vi "Main_Manual_Control.vi"() -> ()   [LabVIEW 2020]
uses:
  States.ctl
  <vilib>/Utility/file.llb/Read Delimited Spreadsheet (I64).vi
  <vilib>/Instr/_visa.llb/VISA Configure Serial Port (Serial Instr).vi
panel:
  in  "Manual Mode":bool
  in  "Tab Control":enum32{"Control", "Debug"}(tab)
  out "Power":dynamicdata(graph)
  in  "Power DAQ":bool
  in  "Log DAQ":bool
  out "Target INC":u16 max=12 step=1
  out "STEP":i32
  out "Target MPH":u16 max=12 step=1
  out "stopping":bool
  in  "Serial Port":refnum<visa-resource-name>="COM8"
  in  "Manual Stop":bool
  in  "TestScript":path=path "C:/LabView Computer Backup SEAL2788/DonP_TRM500/FootTimeInc.txt"
  out "MPH READ":u8
  out "INC READ":u8
  out "PD READ":u8
  out "Speed Changed":bool
  out "Inc Changed":bool
  in  "MPH UP":bool
  in  "MPH DOWN":bool
  in  "INC UP":bool
  in  "INC DOWN":bool
  out "Com Error":errorcluster
  out "Control Error":errorcluster
  out "speed":u16[](array[numeric])
  out "time":u16[](array[numeric])
  out "incline":u16[](array[numeric])
  out "dwell":u16[](array[numeric])
  out "FootPath":path
  out "read buffer":string
  out "Send Buffer":string
  out "Last Speed Sent":string
  out "Last Inc Sent":string
  out "FootPathRef":refnum<file>
  out "input lines":i32
  out "Next Inc":u16
  out "Next Duration":u16
  out "Next MPH":u16
  out "Time Left":u32
  out "Missed Msg":u16
  out "Next Cmd":enum16{"getParm", "inc", "mph", "err"}(ring)
  out "Next Com State":enum16{"Initialize", "Send", "Receive", "Error"}(ring)=enum."Receive"
  out "Next Control State":T1
  # "Control Panel"
  # "Debug Panel"
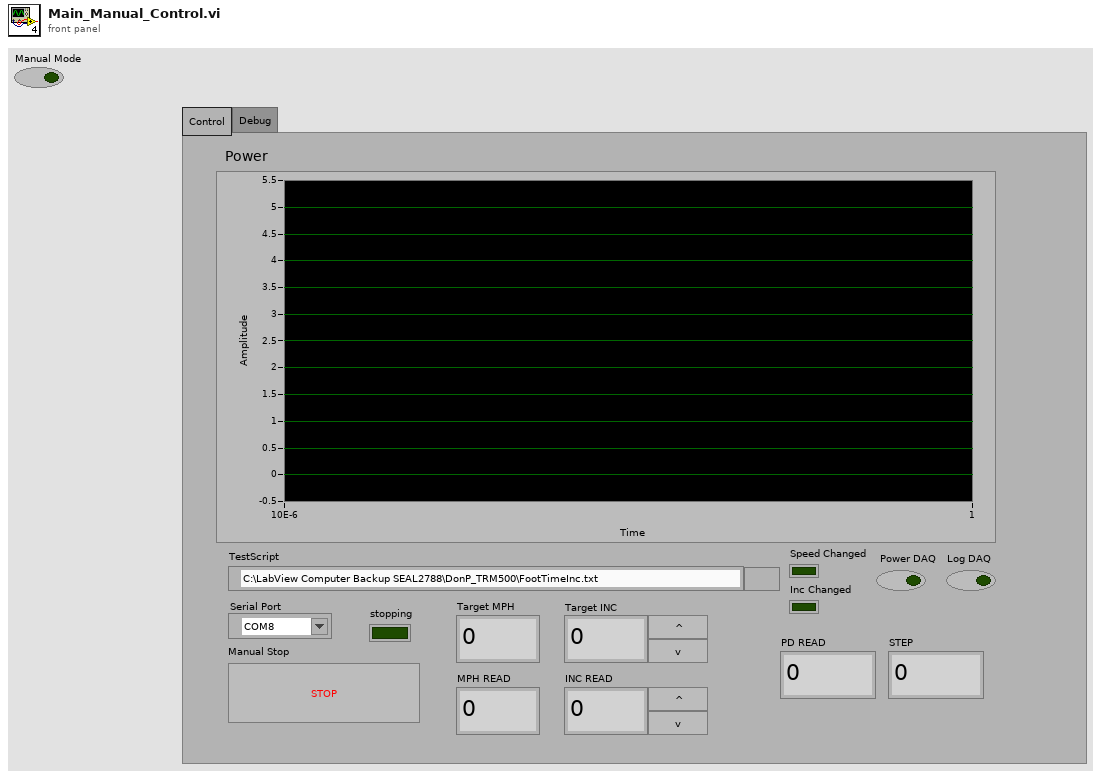
[diagram p1: front panel]
types:
  T1 = typedef "States.ctl" = enum16{"Initialize", "SetTargets", "WaitforMPH", "Dwell", "CheckTiming"}
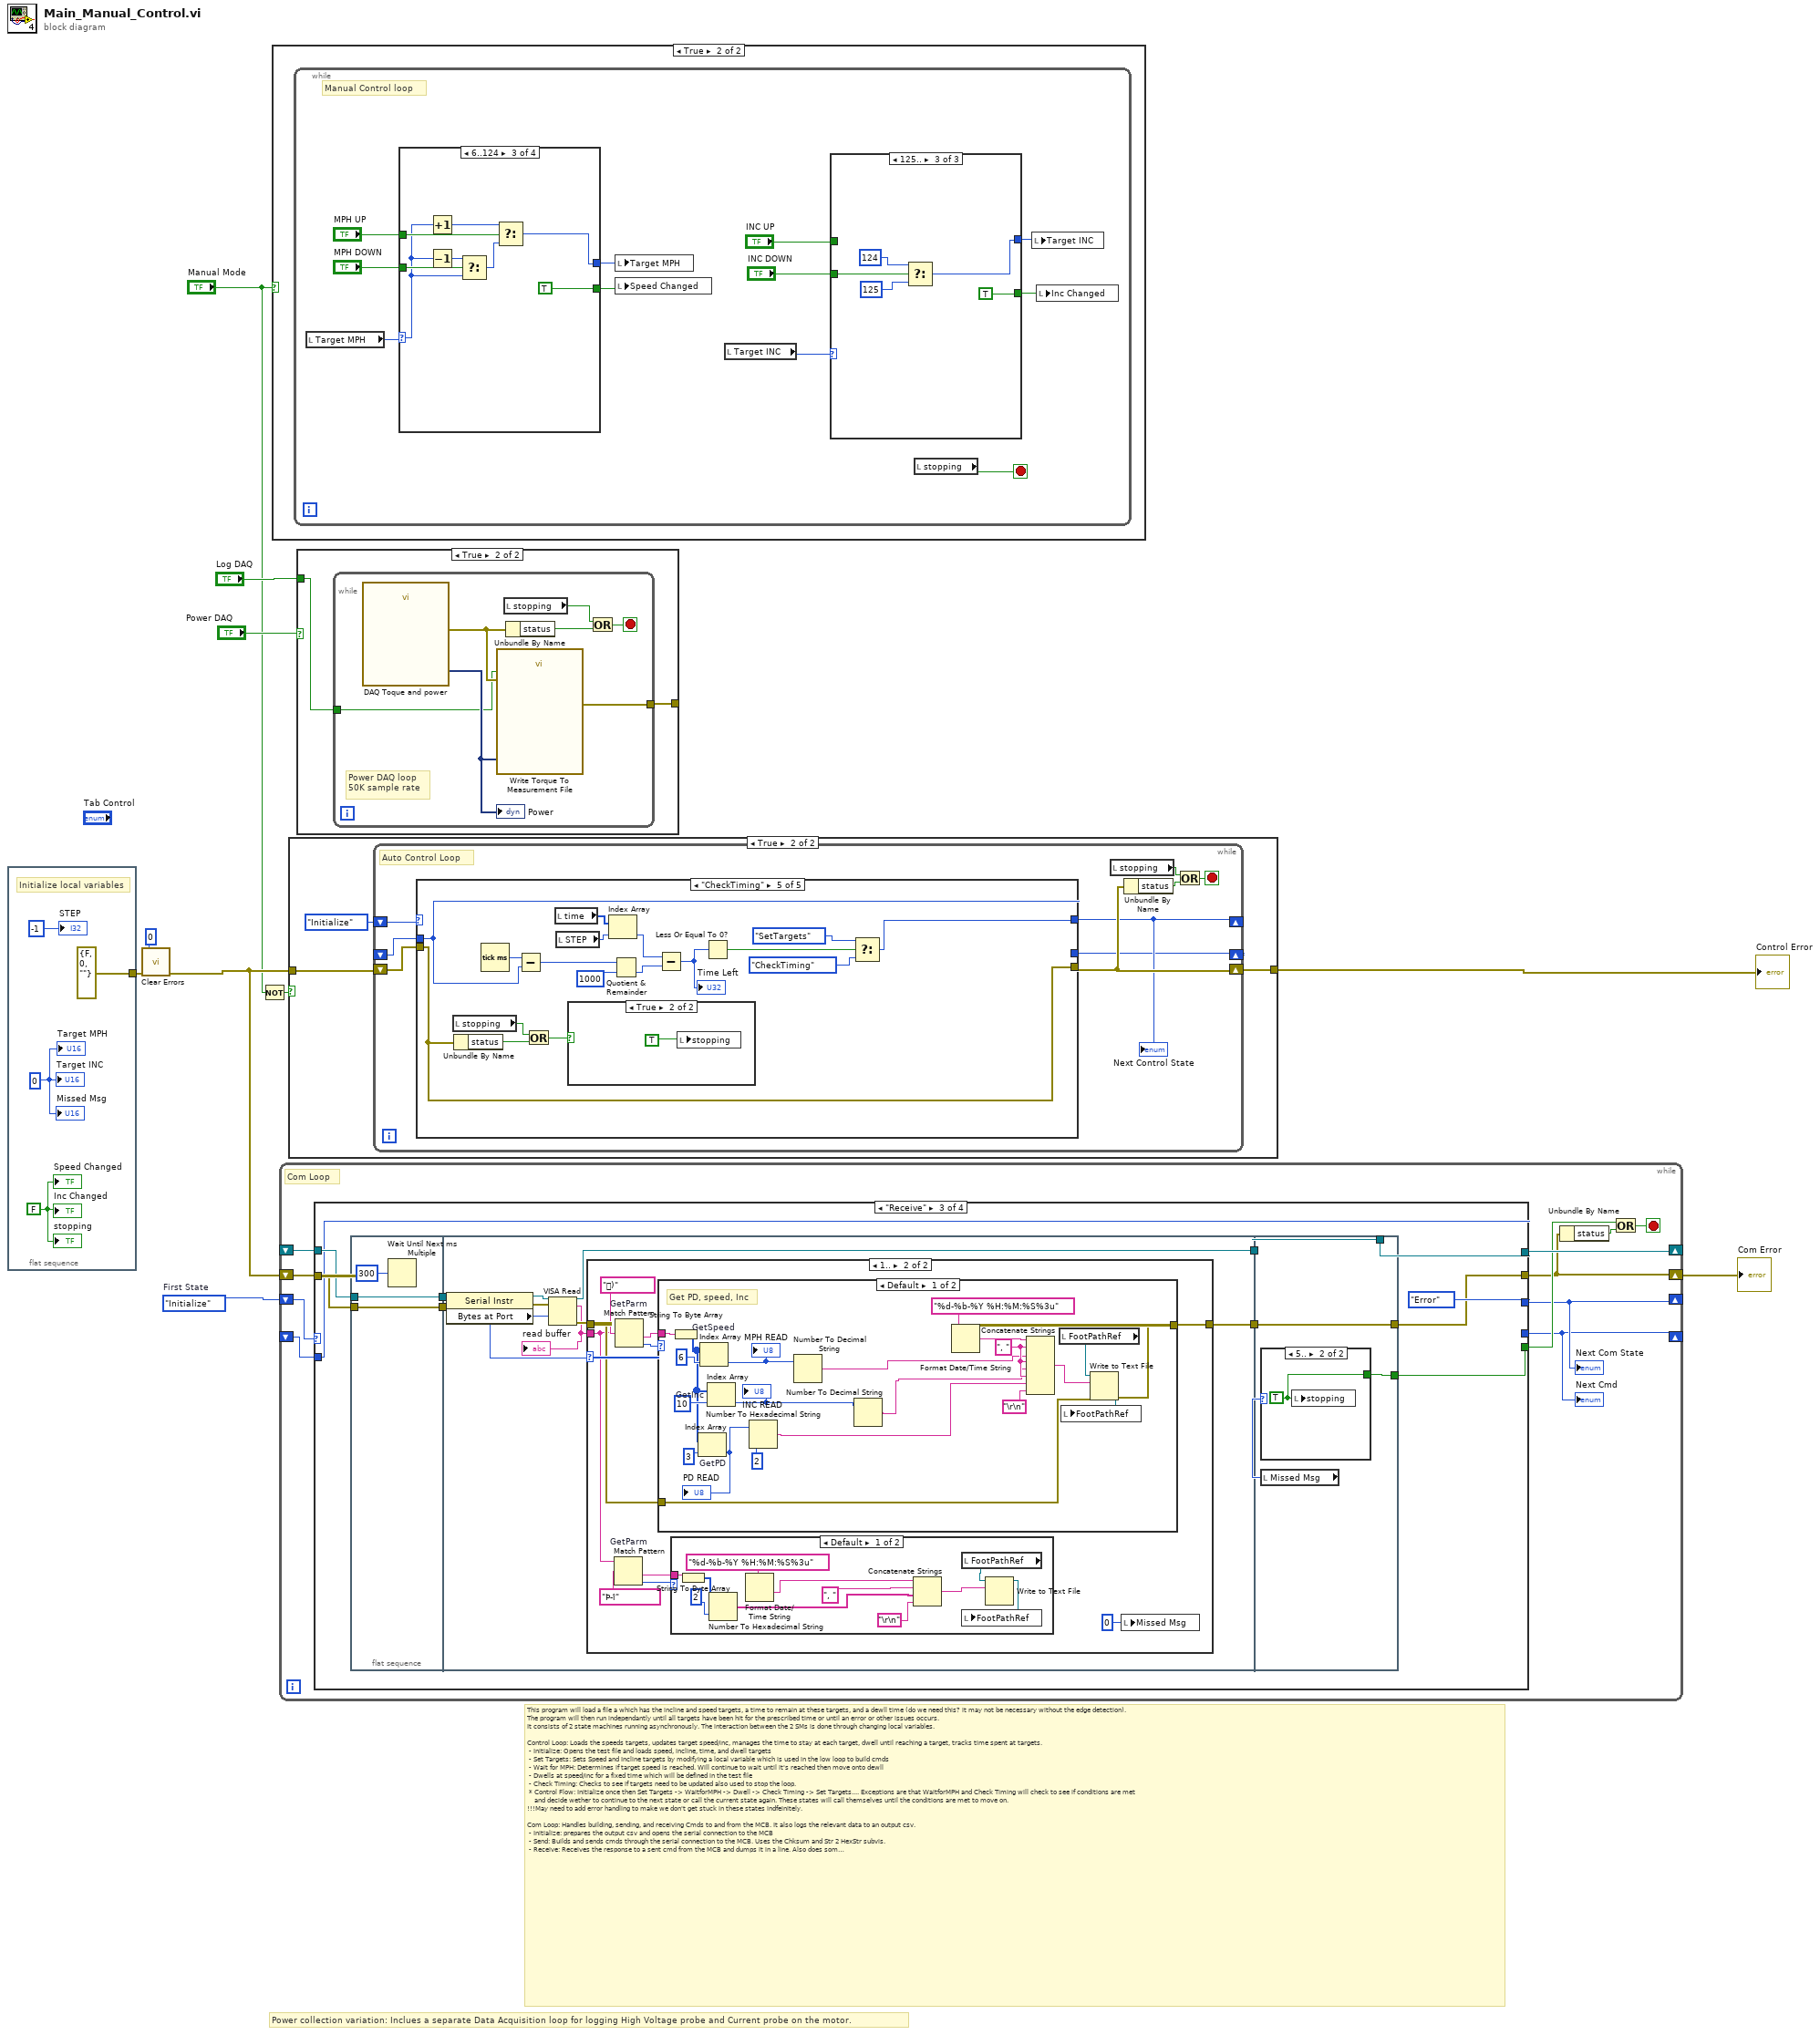
[diagram p0: block diagram]
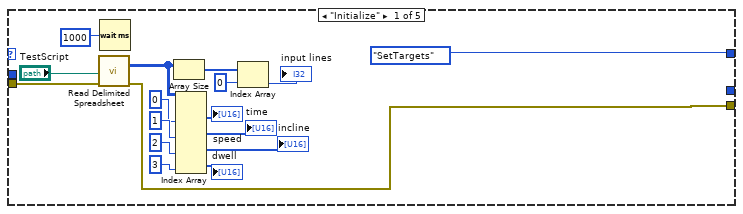
[diagram p3: hidden frame]
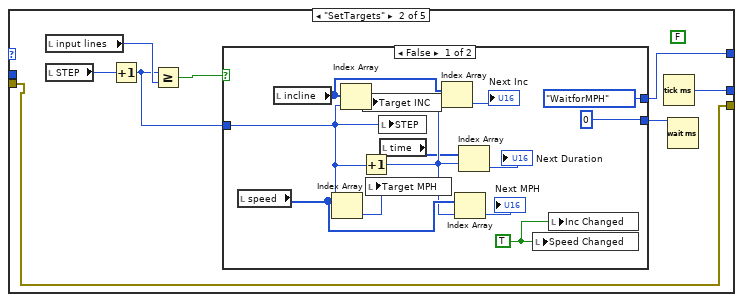
[diagram p4: hidden frame]
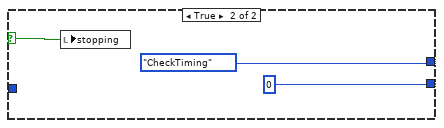
[diagram p5: hidden frame]
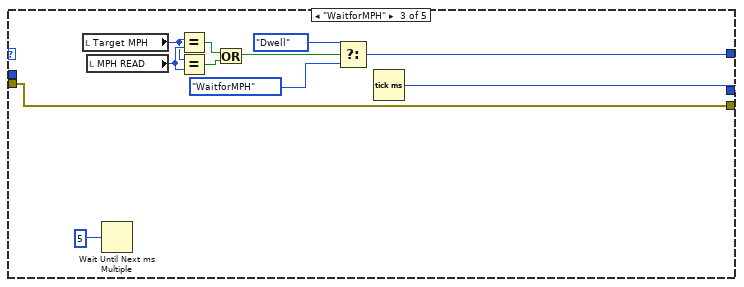
[diagram p6: hidden frame]
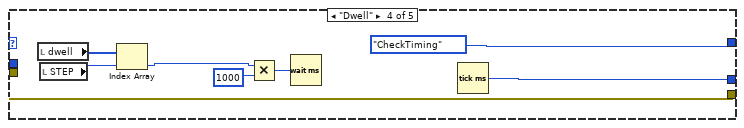
[diagram p7: hidden frame]
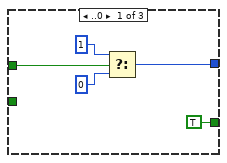
[diagram p10: hidden frame]
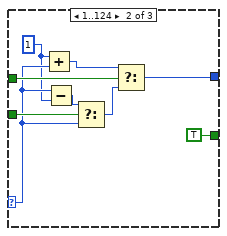
[diagram p11: hidden frame]
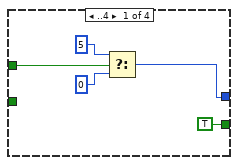
[diagram p12: hidden frame]
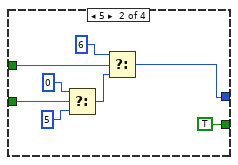
[diagram p13: hidden frame]
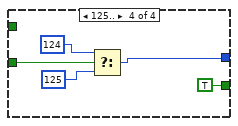
[diagram p14: hidden frame]
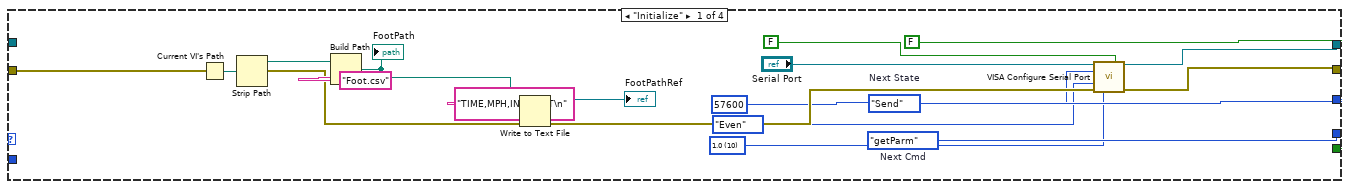
[diagram p16: hidden frame]
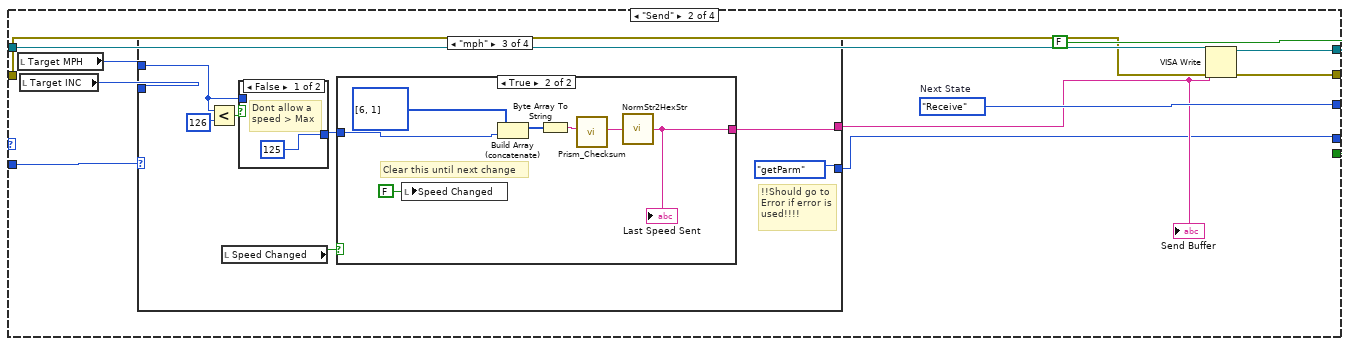
[diagram p17: hidden frame]
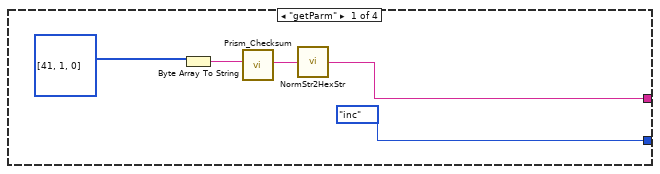
[diagram p18: hidden frame]
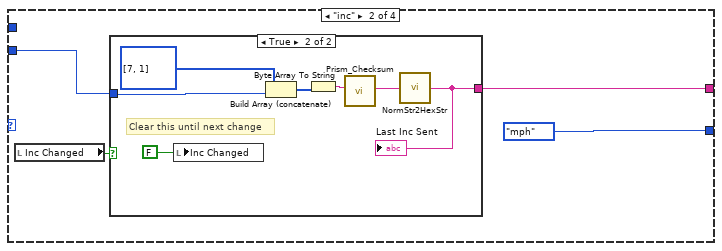
[diagram p19: hidden frame]
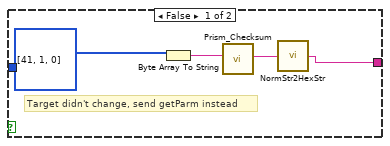
[diagram p20: hidden frame]
diagram:
  w10 = enum16{"Initialize", "Send", "Receive", "Error"}."Initialize"  # First State
  # "Power collection variation: Inclues a separate Data Acquisition loop for logging High Voltage probe and Current probe on the motor."
  # "This program will load a file a which has the incline and speed targets, a time to remain at these targets, and a dewll time (do we need this? it may not be necessary without the edge detection).\nThe program will then run independantly until all targets have been hit for the prescribed time or until an error or other issues occurs.\nIt consists of 2 state machines running asynchronously. The interaction between the 2 SMs is done through changing local variables.\n\nControl Loop: Loads the speeds targets, updates target speed/inc, manages the time to stay at each target, dwell until reaching a target, tracks time spent at targets. \n - Initialize: Opens the test file and loads speed, incline, time, and dwell targets \n - Set Targets: Sets Speed and Incline targets by modifying a local variable which is used in the low loop to build cmds \n - Wait for MPH: Determines if target speed is reached. Will continue to wait until it's reached then move onto dewll\n - Dwells at speed/inc for a fixed time which will be defined in the test file\n - Check Timing: Checks to see if targets need to be updated also used to stop the loop.\n * Control Flow: Initialize once then Set Targets -> WaitforMPH -> Dwell -> Check Timing -> Set Targets.... Exceptions are that WaitforMPH and Check Timing will check to see if conditions are met\n    and decide wether to continue to the next state or call the current state again. These states will call themselves until the conditions are met to move on. \n!!!May need to add error handling to make we don't get stuck in these states indfeinitely.\n\nCom Loop: Handles building, sending, and receiving Cmds to and from the MCB. It also logs the relevant data to an output csv.\n - Initialize: prepares the output csv and opens the serial connection to the MCB\n - Send: Builds and sends cmds through the serial connection to the MCB. Uses the Chksum and Str 2 HexStr subvis. \n - Receive: Receives the response to a sent cmd from the MCB and dumps it in a line. Also does some analysis of the response to determine current  Speed/inc/person detect\n - Error:  Stops the program. This handles labview errors and will stop the program when one is encounted. It also handles stopping when reaching the end of a test \n * Com Flow: nitialize once then Send -> Receive -> Error -> Send...\n * Send flow: GetParm -> Inc -> MPH -> GetParm etc. Exception is that it will check first to see if the target changed and if it hasn't will send getParm Instead\n!!!May need to add error handling in which case the flow should be GetParm -> MPH -> Inc -> Err -> GetParm....\n\nFiles:\n1 input file which contains the test script to run. Format: Speed, Time, Inc, Dwell. Time = time to stay at target speed/inc. Dwell = a fixed time to wait after reaching targets and before starting the Time counter. This is used to make sure the speed stablizes before starting the Time counter.\n1 output file which contains Timestamp, Speed, Incline, and a flag for if person is detected (0 = No, 1 = Yes). Format: TIME,MPH,INC,FOOT"
  n1 = flat-sequence {
    tunnel: [errorcluster {"status"=FALSE, "code"=0, "source"=""} ("error constant")] -> w7
    frame #0 {
      w12 = FALSE ("Inc Changed")
      w11 = u16 0 ("MPH")
      # "Initialize local variables"
      "stopping" <- w12
      "Target MPH" <- w11
      "STEP" <- -1 ("step")
      "Target INC" <- w11
      "Speed Changed" <- w12
      "Inc Changed" <- w12
      "Missed Msg" <- w11
    }
  }
  n2 = call <vilib>:"Clear Errors.vi"("error in (no error)"=w7, "specific error code to clear (0: all)"=0) -> ("error out"=w6:errorcluster)  [unwired: 4 in, 1 out]
  n3 = Not(x="Manual Mode") -> (.not. x?=w1:bool)
  n4 = case shown="True" "Manual Mode" {
    frame False {
    }
    frame True {
      n5 = while {
        stop <- w25 stop-if-true
        # "Manual Control loop"
        n6 = local read "Target MPH"() -> (w20:u16)
        n7 = case shown="6..124" w20 {
          selector: w20 -> [_ _ w61 _]
          tunnel: "MPH UP" -> [w49 w57 w65 _]
          tunnel: "MPH DOWN" -> [_ w54 w63 w70]
          tunnel: [w46 w51 w59 w67] -> w18
          tunnel: [TRUE TRUE TRUE TRUE] -> w16
          frame ..4 {
            n8 = Select(t=5 ("MPH"), s=w49, f=0 ("MPH")) -> (s? t:f=w46:i32)
          }
          frame 5 {
            n9 = Select(t=0 ("MPH"), s=w54, f=5 ("MPH")) -> (s? t:f=w55:i32)
            n10 = Select(t=6 ("MPH"), s=w57, f=w55) -> (s? t:f=w51:i32)
          }
          frame 6..124 {
            n11 = Increment(x=w61) -> (x+1=w60:u16)
            n12 = Decrement(x=w61) -> (x-1=w62:u16)
            n13 = Select(t=w62, s=w63, f=w61) -> (s? t:f=w64:u16)
            n14 = Select(t=w60, s=w65, f=w64) -> (s? t:f=w59:u16)
          }
          frame 125.. {
            n15 = Select(t=124 ("MPH"), s=w70, f=125) -> (s? t:f=w67:i32)
          }
        }
        n16 = local write "Target MPH"(w18) -> ()
        n17 = local write "Speed Changed"(w16) -> ()
        n18 = local read "Target INC"() -> (w19:u16)
        n19 = case shown="125.." w19 {
          selector: w19 -> [_ w35 _]
          tunnel: "INC UP" -> [w30 w39 _]
          tunnel: "INC DOWN" -> [_ w37 w44]
          tunnel: [w27 w32 w41] -> w17
          tunnel: [TRUE TRUE TRUE] -> w15
          frame ..0 {
            n20 = Select(t=1 ("MPH"), s=w30, f=0 ("MPH")) -> (s? t:f=w27:i32)
          }
          frame 1..124 {
            w34 = 1
            n21 = Add(x=w34, y=w35) -> (x+y=w36:i32)
            n22 = Subtract(x=w35, y=w34) -> (x-y=w33:i32)
            n23 = Select(t=w33, s=w37, f=w35) -> (s? t:f=w38:i32)
            n24 = Select(t=w36, s=w39, f=w38) -> (s? t:f=w32:i32)
          }
          frame 125.. {
            n25 = Select(t=124 ("MPH"), s=w44, f=125) -> (s? t:f=w41:i32)
          }
        }
        n26 = local read "stopping"() -> (w25:bool)
        n27 = local write "Target INC"(w17) -> ()
        n28 = local write "Inc Changed"(w15) -> ()
      }
    }
  }
  n29 = while {
    shift-right: [w75] -> w9
    shift-left: w6 -> [w81]
    shift-right: [w78] -> _
    shift-left: _ -> [w80]
    shift-right: [w72] -> _
    shift-left: w10 -> [w79]
    shift-right: [w71] -> _
    shift-left: _ -> [w77]
    stop <- w74 stop-if-true
    # "Com Loop"
    n30 = case shown="\"Receive\"" w79 {
      tunnel: w81 -> [w87 w101 w164 w234]
      tunnel: w80 -> [_ w108 w166 w232]
      tunnel: [w97 w110 w160 w231] -> w78
      tunnel: [w96 w109 w159 w233] -> w75
      tunnel: [w93 w104 enum16{"Initialize", "Send", "Receive", "Error"}."Error" enum16{"Initialize", "Send", "Receive", "Error"}."Send"] -> w72
      tunnel: [w95 w102 w163 w239] -> w71
      tunnel: w77 -> [_ w100 w163 w239]
      tunnel: [FALSE FALSE w156 w235] -> w76
      frame "Initialize" {
        w82 = u16 10 items=["1.0"=10, "1.5"=15, "2.0"=20] ("stop bits (10: 1 bit)")
        w93 = enum16{"Initialize", "Send", "Receive", "Error"}."Send"  # Next State
        w95 = enum16{"getParm", "inc", "mph", "err"}."getParm"  # Next Cmd
        n31 = Current VI's Path() -> (path=w92:path)
        n32 = Strip Path(path=w92) -> (stripped path=w91:path)  [unwired: 1 out]
        n33 = Build Path(base path=w91, name or relative path="Foot.csv") -> (appended path=w88:path)
        "FootPath" <- w88
        n34 = Write to Text File(file (use dialog)=w88, text="TIME,MPH,INC,FOOT\n", error in=w87) -> (refnum out=→"FootPathRef":refnum<file>, error out=w86:errorcluster)  [unwired: 1 in, 1 out]
        n35 = call-poly "VISA Configure Serial Port"("VISA resource name"="Serial Port", "Enable Termination\nChar (T)"=FALSE ("Enable Termination\nChar (T)"), "baud rate (9600)"=u32 57600, "parity (0:none)"=enum16{"None", "Odd", "Even", "Mark", "Space"}."Even", "error in (no error)"=w86, "stop bits (10: 1 bit)"=w82) -> ("VISA resource name out"=w97:refnum<visa-resource-name>, "error out"=w96:errorcluster)  [unwired: 8 in]
      }
      frame "Send" {
        w104 = enum16{"Initialize", "Send", "Receive", "Error"}."Receive"  # Next State
        n36 = local read "Target MPH"() -> (w106:u16)
        n37 = local read "Target INC"() -> (w105:u16)
        n38 = case shown="\"mph\"" w100 {
          tunnel: w106 -> [_ _ w132 _]
          tunnel: w105 -> [_ w119 _ _]
          tunnel: [w111 w118 w136 w152] -> w103
          tunnel: [enum16{"getParm", "inc", "mph", "err"}."inc" enum16{"getParm", "inc", "mph", "err"}."mph" enum16{"getParm", "inc", "mph", "err"}."getParm" enum16{"getParm", "inc", "mph", "err"}."getParm"] -> w102
          frame "getParm" {
            n39 = Byte Array To String(unsigned byte array=u8[] [41, 1, 0]) -> (string=w113:string)
            n40 = call "Prism_Checksum.vi"("ID +DB+ Data"=w113) -> ("Full Cmd"=w112:string)  [unwired: 10 in]
            n41 = call "NormStr2HexStr.vi"("string"=w112) -> ("hex string"=w111:string)
          }
          frame "inc" {
            n42 = local read "Inc Changed"() -> (w116:bool)
            n43 = case shown="True" w116 {
              tunnel: w119 -> [_ w127]
              tunnel: [w120 w125] -> w118
              frame False {
                # "Target didn't change, send getParm instead"
                n44 = Byte Array To String(unsigned byte array=u8[] [41, 1, 0]) -> (string=w122:string)
                n45 = call "Prism_Checksum.vi"("ID +DB+ Data"=w122) -> ("Full Cmd"=w121:string)  [unwired: 10 in]
                n46 = call "NormStr2HexStr.vi"("string"=w121) -> ("hex string"=w120:string)
              }
              frame True {
                # "Clear this until next change"
                n47 = local write "Inc Changed"(FALSE ("Value Changed")) -> ()
                n48 = Build Array (concatenate)(u8[] [7, 1] ("unsigned byte array"), w127) -> (w126:u16[])
                n49 = Byte Array To String(unsigned byte array=w126) -> (string=w129:string)
                n50 = call "Prism_Checksum.vi"("ID +DB+ Data"=w129) -> ("Full Cmd"=w130:string)  [unwired: 10 in]
                n51 = call "NormStr2HexStr.vi"("string"=w130) -> ("hex string"=w125:string)
                "Last Inc Sent" <- w125
              }
            }
          }
          frame "mph" {
            # "!!Should go to\nError if error is\nused!!!!"
            n52 = Less?(x=w132, y=u16 126) -> (x < y?=w134:bool)
            n53 = local read "Speed Changed"() -> (w135:bool)
            n54 = case shown="False" w134 {
              tunnel: w132 -> [_ w139]
              tunnel: [u16 125 ("Target MPH") w139] -> w131
              frame False {
                # "Dont allow a\nspeed > Max"
              }
              frame True {
              }
            }
            n55 = case shown="True" w135 {
              tunnel: [w140 w147] -> w136
              tunnel: w131 -> [_ w145]
              frame False {
                # "Target didn't change, send getParm instead"
                n56 = Byte Array To String(unsigned byte array=u8[] [41, 1, 0]) -> (string=w142:string)
                n57 = call "Prism_Checksum.vi"("ID +DB+ Data"=w142) -> ("Full Cmd"=w141:string)  [unwired: 10 in]
                n58 = call "NormStr2HexStr.vi"("string"=w141) -> ("hex string"=w140:string)
              }
              frame True {
                # "Clear this until next change"
                n59 = local write "Speed Changed"(FALSE ("Value Changed")) -> ()
                n60 = Build Array (concatenate)(u8[] [6, 1] ("unsigned byte array"), w145) -> (w146:u16[])
                n61 = Byte Array To String(unsigned byte array=w146) -> (string=w149:string)
                n62 = call "Prism_Checksum.vi"("ID +DB+ Data"=w149) -> ("Full Cmd"=w150:string)  [unwired: 10 in]
                n63 = call "NormStr2HexStr.vi"("string"=w150) -> ("hex string"=w147:string)
                "Last Speed Sent" <- w147
              }
            }
          }
          frame "err" {
            # "!!Not in used currently. DELETE this if implemented!!!"
            # "!!!!Add logic to\nhandle/ clear erros!!!!!!"
            n64 = Byte Array To String(unsigned byte array=u8[] [30, 1, 0]) -> (string=w154:string)
            n65 = call "Prism_Checksum.vi"("ID +DB+ Data"=w154) -> ("Full Cmd"=w155:string)  [unwired: 10 in]
            n66 = call "NormStr2HexStr.vi"("string"=w155) -> ("hex string"=w152:string)
          }
        }
        "Send Buffer" <- w103
        n67 = VISA Write(VISA resource name=w108, write buffer=w103, error in (no error)=w101) -> (VISA resource name out=w110:refnum<visa-resource-name>, error out=w109:errorcluster)  [unwired: 1 out]
      }
      frame "Receive" {
        n68 = flat-sequence {
          tunnel: w166 -> [w168]
          tunnel: w164 -> [w167]
          tunnel: [w168] -> w162
          tunnel: [w167] -> w161
          tunnel: w162 -> [w178]
          tunnel: w161 -> [w177]
          tunnel: [w170] -> w158
          tunnel: [w174] -> w157
          tunnel: [w227] -> w159
          tunnel: [w228] -> w160
          tunnel: w158 -> [w228]
          tunnel: w157 -> [w227]
          tunnel: [w225] -> w156
          frame #0 {
            n69 = Wait Until Next ms Multiple(millisecond multiple=u32 300) -> ()  [unwired: 1 out]
          }
          frame #1 {
            n70 = property class="Serial Instr"(reference=w178, error in=w177) -> (reference out=w175:refnum<visa-resource-name>, error out=w176:errorcluster, "Bytes at Port"=w173:u32)
            n71 = VISA Read(VISA resource name=w175, byte count=w173, error in (no error)=w176) -> (VISA resource name out=w170:refnum<visa-resource-name>, read buffer=w171:string, error out=w172:errorcluster)  [unwired: 1 out]
            "read buffer" <- w171
            n72 = case shown="1.." w173 {
              tunnel: [w181 w188] -> w174
              tunnel: w172 -> [w181 w187]
              tunnel: w171 -> [_ w186]
              frame 0 {
                n73 = local read "Missed Msg"() -> (w180:u16)
                n74 = Increment(x=w180) -> (x+1=w179:u16)
                n75 = local write "Missed Msg"(w179) -> ()
              }
              frame 1.. {
                n76 = Match Pattern "GetParm"(string=w186, regular expression="Þ­î") -> (after substring=w183:string, offset past match=w184:i32)  [unwired: 1 in, 2 out]
                n77 = Match Pattern "GetParm"(string=w186, regular expression="ޭ)") -> (after substring=w190:string, offset past match=w189:i32)  [unwired: 1 in, 2 out]
                n78 = case shown="Default" w189 {
                  tunnel: w190 -> [w204 _]
                  tunnel: [w217 w224] -> w188
                  tunnel: w187 -> [w212 w224]
                  frame Default {
                    w211 = ", "
                    # "Get PD, speed, Inc"
                    n79 = String To Byte Array(string=w204) -> (unsigned byte array=w220:u8[])
                    n80 = Index Array "GetPD"(array=w220, index=3) -> (element=w214:u8)
                    "PD READ" <- w214
                    n81 = Index Array "GetSpeed"(array=w220, index=6) -> (element=w206:u8)
                    "MPH READ" <- w206
                    n82 = Index Array "GetInc"(array=w220, index=10) -> (element=w205:u8)
                    "INC READ" <- w205
                    n83 = Number To Hexadecimal String(1:i16 2 ("width (-)"), 2:w214) -> (0:w209:string)
                    n84 = Number To Decimal String(number=w206) -> (decimal integer string=w208:string)  [unwired: 1 in]
                    n85 = Number To Decimal String(number=w205) -> (decimal integer string=w207:string)  [unwired: 1 in]
                    n86 = Format Date/Time String(time format string (%c)="%d-%b-%Y %H:%M:%S%3u") -> (date/time string=w215:string)  [unwired: 2 in]
                    n87 = Concatenate Strings(w215, w211, w208, w211, w207, w211, w209, "\r\n") -> (w218:string)
                    n88 = local read "FootPathRef"() -> (w216:refnum<file>)
                    n89 = Write to Text File(file (use dialog)=w216, text=w218, error in=w212) -> (refnum out=w210:refnum<file>, error out=w217:errorcluster)  [unwired: 1 in, 1 out]
                    n90 = local write "FootPathRef"(w210) -> ()
                  }
                  frame -1 {
                  }
                }
                n91 = case shown="Default" w184 {
                  tunnel: w183 -> [w197 _]
                  frame Default {
                    n92 = String To Byte Array(string=w197) -> (unsigned byte array=w195:u8[])
                    n93 = Number To Hexadecimal String(1:i16 2 ("width (-)"), 2:w195) -> (0:w192:string[])
                    n94 = Format Date/Time String(time format string (%c)="%d-%b-%Y %H:%M:%S%3u") -> (date/time string=w199:string)  [unwired: 2 in]
                    n95 = Concatenate Strings(w199, ", ", w192, "\r\n") -> (w198:string)
                    n96 = local read "FootPathRef"() -> (w202:refnum<file>)
                    n97 = Write to Text File(file (use dialog)=w202, text=w198) -> (refnum out=w201:refnum<file>)  [unwired: 2 in, 2 out]
                    n98 = local write "FootPathRef"(w201) -> ()
                  }
                  frame -1 {
                  }
                }
                n99 = local write "Missed Msg"(u16 0 ("Missed Msg")) -> ()
              }
            }
          }
          frame #2 {
            n100 = local read "Missed Msg"() -> (w226:u16)
            n101 = case shown="5.." w226 {
              tunnel: [FALSE ("stopping") w230] -> w225
              frame ..4 {
              }
              frame 5.. {
                w230 = TRUE ("stopping")
                n102 = local write "stopping"(w230) -> ()
              }
            }
          }
        }
      }
      frame "Error" {
        n103 = local read "stopping"() -> (w236:bool)
        n104 = Compound Arithmetic op=OR("Manual Stop", w236, w234) -> (w238:bool)
        n105 = case shown="True" w238 {
          tunnel: [FALSE w244] -> w235
          tunnel: w234 -> [w242 w252]
          tunnel: [w242 w251] -> w233
          tunnel: w232 -> [w241 w250]
          tunnel: [w241 w249] -> w231
          frame False {
          }
          frame True {
            n106 = flat-sequence {
              tunnel: w252 -> [w256]
              tunnel: w250 -> [w254]
              tunnel: [w255] -> w248
              tunnel: [w253] -> w247
              tunnel: w248 -> [w263]
              tunnel: w247 -> [w262]
              tunnel: [w263] -> w246
              tunnel: [w262] -> w245
              tunnel: [w265] -> w249
              tunnel: [w264] -> w251
              tunnel: w246 -> [w266]
              tunnel: w245 -> [w267]
              tunnel: [w272] -> w244
              frame #0 {
                # "Stopping so send 0 MPH first"
                n107 = Byte Array To String(unsigned byte array=u8[] [6, 1, 0]) -> (string=w260:string)
                n108 = call "Prism_Checksum.vi"("ID +DB+ Data"=w260) -> ("Full Cmd"=w259:string)  [unwired: 10 in]
                n109 = call "NormStr2HexStr.vi"("string"=w259) -> ("hex string"=w258:string)
                n110 = VISA Write(VISA resource name=w254, write buffer=w258, error in (no error)=w256) -> (VISA resource name out=w253:refnum<visa-resource-name>, error out=w255:errorcluster)  [unwired: 1 out]
              }
              frame #1 {
                # "Wait..."
                n111 = Wait (ms)(milliseconds to wait=u32 100) -> ()  [unwired: 1 out]
              }
              frame #2 {
                w272 = TRUE ("stopping")
                # "Stopping so send 0 inc first"
                n112 = Byte Array To String(unsigned byte array=u8[] [7, 1, 0]) -> (string=w271:string)
                n113 = call "Prism_Checksum.vi"("ID +DB+ Data"=w271) -> ("Full Cmd"=w270:string)  [unwired: 10 in]
                n114 = local write "stopping"(w272) -> ()
                n115 = call "NormStr2HexStr.vi"("string"=w270) -> ("hex string"=w269:string)
                n116 = VISA Write(VISA resource name=w267, write buffer=w269, error in (no error)=w266) -> (VISA resource name out=w265:refnum<visa-resource-name>, error out=w264:errorcluster)  [unwired: 1 out]
              }
            }
          }
        }
      }
    }
    "Next Com State" <- w72
    "Next Cmd" <- w71
    n117 = Unbundle By Name(w75) -> ("status"=w73:bool)
    n118 = Or(x=w76, y=w73) -> (x .or. y?=w74:bool)
  }
  "Com Error" <- w9
  n119 = case shown="True" w1 {
    tunnel: [w273 w276] -> w8
    tunnel: w6 -> [w273 w274]
    frame False {
    }
    frame True {
      n120 = while {
        shift-right: [w282] -> w276
        shift-left: w274 -> [w285]
        shift-right: [w280] -> _
        shift-left: _ -> [w279]
        shift-right: [w281] -> _
        shift-left: States."Initialize" ("First State") -> [w278]
        stop <- w283 stop-if-true
        # "Auto Control Loop"
        n121 = case shown="\"CheckTiming\"" w278 {
          tunnel: w285 -> [w300 w303 w336 w342 w346]
          tunnel: [w290 w303 w336 w342 w346] -> w282
          tunnel: [States."SetTargets" ("First State") w307 w334 States."CheckTiming" ("First State") w347] -> w281
          tunnel: [_ w305 w335 w339 w358] -> w280
          tunnel: w279 -> [_ _ _ _ w358]
          frame "Initialize" {
            n122 = call-poly <vilib>:"Read Delimited Spreadsheet.vi"("file path (dialog if empty)"="TestScript", "error in (no error)"=w300) -> ("all rows"=w296:i64[][], "error out"=w290:errorcluster)  [unwired: 8 in, 4 out]
            n123 = Wait (ms)(milliseconds to wait=u32 1000) -> ()  [unwired: 1 out]
            n124 = Array Size(array=w296) -> (size(s)=w298:i32[])
            n125 = Index Array(array=w296, index (col) #1=0 ("index"), index (col) #2=1 ("index (col)"), index (col) #3=2 ("index (col)"), index (col) #4=3 ("index (col)")) -> (element #1=→"speed":i64[], element #2=→"time":i64[], element #3=→"incline":i64[], element #4=→"dwell":i64[])  [unwired: 4 in]
            n126 = Index Array(array=w298, index=0) -> (element=→"input lines":i32)
          }
          frame "SetTargets" {
            (unwired) FALSE
            n127 = local read "input lines"() -> (w309:i32)
            n128 = local read "STEP"() -> (w310:i32)
            n129 = Increment(x=w310) -> (x+1=w304:i32)
            n130 = Greater Or Equal?(x=w304, y=w309) -> (x >= y?=w308:bool)
            n131 = case shown="False" w308 {
              selector: w308 -> [_ w326]
              tunnel: [States."WaitforMPH" ("First State") States."CheckTiming" ("First State")] -> w307
              tunnel: [u32 0 ("milliseconds to wait") u32 0 ("milliseconds to wait")] -> w306
              tunnel: w304 -> [w321 _]
              frame False {
                w312 = TRUE ("Value Changed")
                n132 = local read "speed"() -> (w320:u16[])
                n133 = local read "incline"() -> (w319:u16[])
                n134 = Index Array(array=w320, index=w321) -> (element=w323:u16)
                n135 = Index Array(array=w319, index=w321) -> (element=w322:u16)
                n136 = Increment(x=w321) -> (x+1=w318:i32)
                n137 = local write "Target INC"(w322) -> ()
                n138 = local write "Target MPH"(w323) -> ()
                n139 = local write "STEP"(w321) -> ()
                n140 = local read "time"() -> (w317:u16[])
                n141 = Index Array(array=w319, index=w318) -> (element=→"Next Inc":u16)
                n142 = Index Array(array=w320, index=w318) -> (element=→"Next MPH":u16)
                n143 = Index Array(array=w317, index=w318) -> (element=→"Next Duration":u16)
                n144 = local write "Speed Changed"(w312) -> ()
                n145 = local write "Inc Changed"(w312) -> ()
              }
              frame True {
                n146 = local write "stopping"(w326) -> ()
              }
            }
            n147 = Tick Count (ms)() -> (millisecond timer value=w305:u32)
            n148 = Wait (ms)(milliseconds to wait=w306) -> ()  [unwired: 1 out]
          }
          frame "WaitforMPH" {
            n149 = local read "Target MPH"() -> (w329:u16)
            n150 = local read "MPH READ"() -> (w330:u8)
            n151 = Wait Until Next ms Multiple(millisecond multiple=u32 5) -> ()  [unwired: 1 out]
            n152 = Equal?(x=w329, y=w330) -> (x = y?=w332:bool)
            n153 = Equal?(x=w329, y=w330) -> (x = y?=w331:bool)
            n154 = Or(x=w332, y=w331) -> (x .or. y?=w333:bool)
            n155 = Select(t=States."Dwell" ("First State"), s=w333, f=States."WaitforMPH" ("First State")) -> (s? t:f=w334:T1)
            n156 = Tick Count (ms)() -> (millisecond timer value=w335:u32)
          }
          frame "Dwell" {
            n157 = local read "dwell"() -> (w340:u16[])
            n158 = local read "STEP"() -> (w341:i32)
            n159 = Index Array(array=w340, index=w341) -> (element=w345:u16)
            n160 = Multiply(x=w345, y=u16 1000) -> (x*y=w343:u16)
            n161 = Wait (ms)(milliseconds to wait=w343) -> ()  [unwired: 1 out]
            n162 = Tick Count (ms)() -> (millisecond timer value=w339:u32)
          }
          frame "CheckTiming" {
            n163 = local read "stopping"() -> (w360:bool)
            n164 = Unbundle By Name(w346) -> ("status"=w361:bool)
            n165 = Tick Count (ms)() -> (millisecond timer value=w362:u32)
            n166 = Subtract(x=w362, y=w358) -> (x-y=w357:u32)
            n167 = Or(x=w360, y=w361) -> (x .or. y?=w359:bool)
            n168 = local read "time"() -> (w355:u16[])
            n169 = local read "STEP"() -> (w354:i32)
            n170 = case shown="True" w359 {
              frame False {
              }
              frame True {
                n171 = local write "stopping"(TRUE ("stopping")) -> ()
              }
            }
            n172 = Index Array(array=w355, index=w354) -> (element=w352:u16)
            n173 = Quotient & Remainder(x=w357, y=u32 1000) -> (floor(x/y)=w353:u32)  [unwired: 1 out]
            n174 = Subtract(x=w352, y=w353) -> (x-y=w351:u32)
            "Time Left" <- w351
            n175 = Less Or Equal To 0?(x=w351) -> (x <= 0?=w350:bool)
            n176 = Select(t=States."SetTargets" ("First State"), s=w350, f=States."CheckTiming" ("First State")) -> (s? t:f=w347:T1)
          }
        }
        "Next Control State" <- w281
        n177 = local read "stopping"() -> (w277:bool)
        n178 = Unbundle By Name(w282) -> ("status"=w284:bool)
        n179 = Or(x=w277, y=w284) -> (x .or. y?=w283:bool)
      }
    }
  }
  "Control Error" <- w8
  n180 = case shown="True" "Power DAQ" {
    tunnel: [_ w365] -> _
    tunnel: "Log DAQ" -> [_ w364]
    frame False {
    }
    frame True {
      n181 = while {
        tunnel: [w369] -> w365
        tunnel: w364 -> [w366]
        stop <- w371 stop-if-true
        # "Power DAQ loop\n50K sample rate"
        n182 = call "DAQ Toque and power"() -> ("data"=w367:dynamicdata, "error out"=w370:errorcluster)  [unwired: 16 in, 2 out]
        "Power" <- w367
        n183 = call "Write Torque To Measurement File"("Signals"=w367, "Enable"=w366, "error in (no error)"=w370) -> ("error out"=w369:errorcluster)  [unwired: 14 in, 2 out]
        n184 = local read "stopping"() -> (w368:bool)
        n185 = Unbundle By Name(w370) -> ("status"=w372:bool)
        n186 = Or(x=w368, y=w372) -> (x .or. y?=w371:bool)
      }
    }
  }
